vi "user32_SetFocus.vi"(0 "hWnd":u32, 11 "错误输入（无错误）":errorcluster) -> (4 "dup hWnd":u32, 6 "success?":bool, 8 "hWnd(old)":u32, 15 "错误输出":errorcluster)   [LabVIEW 2011]
doc: "该函数对指定的窗口设置键盘焦点。该窗口必须与调用线程的消息队列相关。"
uses:
  user32.dll
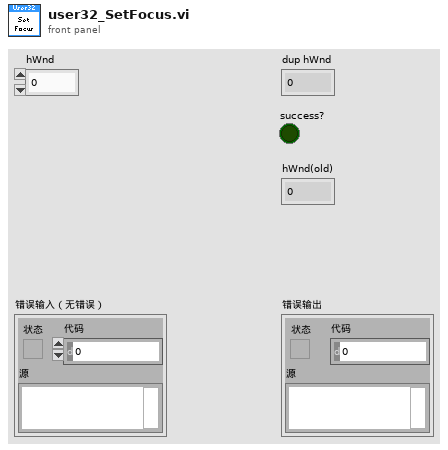
[diagram p1: front panel]
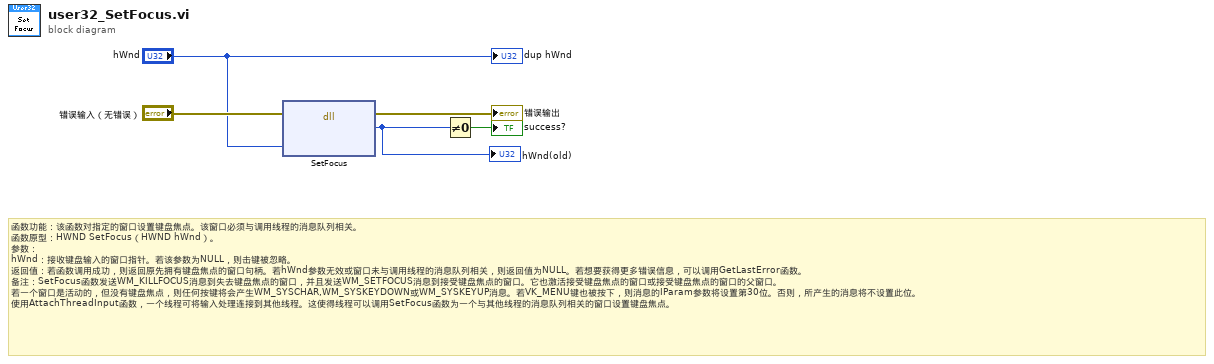
[diagram p0: block diagram]
diagram:
  # "函数功能：该函数对指定的窗口设置键盘焦点。该窗口必须与调用线程的消息队列相关。\n函数原型：HWND SetFocus（HWND hWnd）。\n参数：\nhWnd：接收键盘输入的窗口指针。若该参数为NULL，则击键被忽略。\n返回值：若函数调用成功，则返回原先拥有键盘焦点的窗口句柄。若hWnd参数无效或窗口未与调用线程的消息队列相关，则返回值为NULL。若想要获得更多错误信息，可以调用GetLastError函数。\n备注：SetFocus函数发送WM_KILLFOCUS消息到失去键盘焦点的窗口，并且发送WM_SETFOCUS消息到接受键盘焦点的窗口。它也激活接受键盘焦点的窗口或接受键盘焦点的窗口的父窗口。\n若一个窗口是活动的，但没有键盘焦点，则任何按键将会产生WM_SYSCHAR,WM_SYSKEYDOWN或WM_SYSKEYUP消息。若VK_MENU键也被按下，则消息的IParam参数将设置第30位。否则，所产生的消息将不设置此位。\n使用AttachThreadInput函数，一个线程可将输入处理连接到其他线程。这使得线程可以调用SetFocus函数为一个与其他线程的消息队列相关的窗口设置键盘焦点。"
  n1 = dll-call lib="user32.dll" fn="SetFocus"(error in="错误输入（无错误）", "hWnd"="hWnd") -> (error out=→"错误输出":errorcluster, "hWnd(old)"=w2:u32)  [unwired: 3 in, 1 out]
  "hWnd(old)" <- w2
  n2 = Not Equal To 0?(x=w2) -> (x != 0?=→"success?":bool)
  "dup hWnd" <- "hWnd"
